vi "to_variant_MOVE_MOTION_cmd_data.vi"(10 "target pos":dbl, 11 "OneMotion.lvclass":refnum<class "OneMotion.lvclass">) -> (3 "variant":variant)   [LabVIEW 2016, in "MotionControl_UFO_3DOF.lvlib"]
uses:
  <userlib>/MotionControl_UFO_3DOF/MotionControl_UFO_3DOF.lvlib
  <userlib>/MotionControl_UFO_3DOF/OneMotion/OneMotion.lvclass
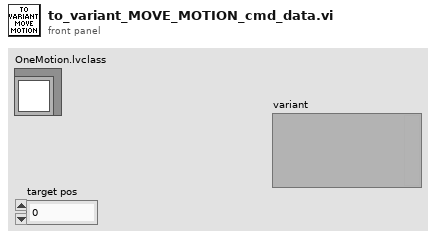
[diagram p1: front panel]
types:
  T1 = cluster{"OneMotion.lvclass":refnum<class "OneMotion.lvclass">, "target pos":dbl}
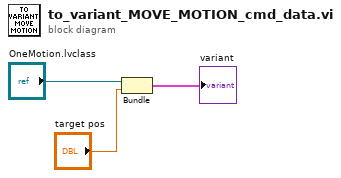
[diagram p0: block diagram]
diagram:
  n1 = Bundle("OneMotion.lvclass"="OneMotion.lvclass", "target pos"="target pos") -> (→"variant":T1)  [unwired: 1 in]
